vi "Set Timeout.vi"(8 "error in (no error)":errorcluster, 10 "Elapsed Time":u32, 11 "Abstract UUT in":refnum<class "Abstract UUT.lvclass">) -> (0 "error out":errorcluster, 2 "Timeout":bool, 3 "Abstract UUT out":refnum<class "Abstract UUT.lvclass">)   [LabVIEW 2019, in "Sequence Main.lvlib" / "Abstract UUT.lvclass"]
uses:
  Abstract UUT.lvclass
  Abstract UUT.lvclass/Abstract UUT.ctl
  <vilib>/addons/TestStand/_TSUtility.llb/TestStand - Get Property Value (Number {Unsigned 32-bit Integer}).vi
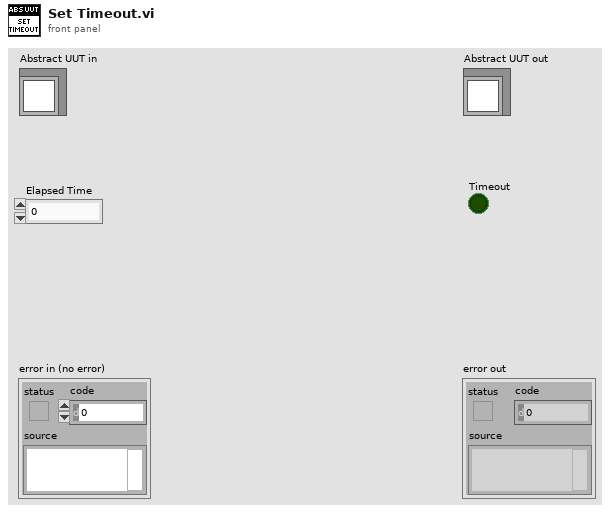
[diagram p1: front panel]
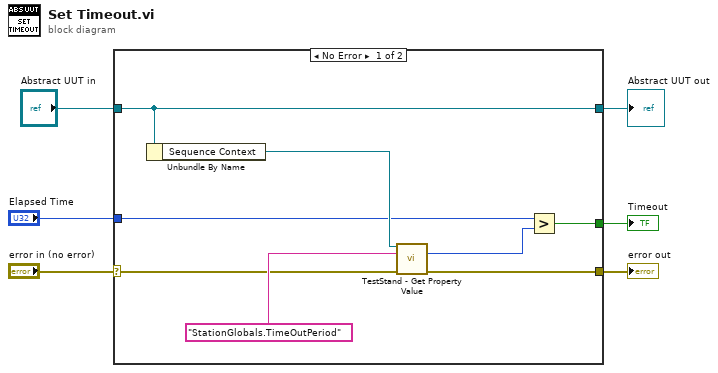
[diagram p0: block diagram]
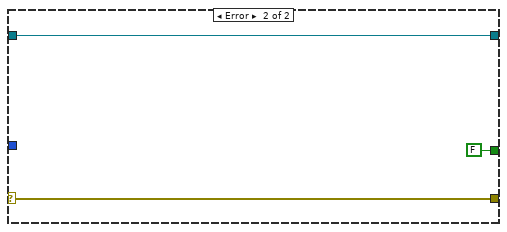
[diagram p2: hidden frame]
diagram:
  n1 = case shown="No Error" "error in (no error)" {
    selector: "error in (no error)" -> [w11 w17]
    tunnel: [w7 w17] -> w5
    tunnel: [w13 w16] -> w3
    tunnel: "Abstract UUT in" -> [w13 w16]
    tunnel: "Elapsed Time" -> [w10 _]
    tunnel: [w8 FALSE] -> w1
    frame No Error {
      n2 = Unbundle By Name(w13) -> ("Sequence Context"=w12:refnum<k7>)
      n3 = call-poly <vilib>:"TestStand - Get Property Value.vi"("Sequence Context In"=w12, "Lookup String"="StationGlobals.TimeOutPeriod", "error in (no error)"=w11) -> ("Value"=w9:u32, "error out"=w7:errorcluster)  [unwired: 10 in, 1 out]
      n4 = Greater?(x=w10, y=w9) -> (0:w8:bool)
    }
    frame Error {
    }
  }
  "error out" <- w5
  "Abstract UUT out" <- w3
  "Timeout" <- w1
